vi "Config Input Settings.vi"(0 "VISA resource name":refnum<visa-resource-name>, 5 "Input (0: A)":u16(ring) items=["A", "B", "C", "D"], 7 "Compensation (0: Off)":i8(ring) items=["Off", "On", "Pause", "Reverse"], 9 "Scan Enable (F: Disable Scanning)":bool, 11 "error in (no error)":errorcluster, 12 "Curve Number (0)":dbl min=0.0 max=60.0 step=1.0) -> (4 "VISA resource name out":refnum<visa-resource-name>, 15 "error out":errorcluster)   [LabVIEW 2019, in "Lake Shore Cryotronics 340.lvlib"]
doc: "This VI configures the following settings for the 340 inputs:\nScan Enable, Compensation, and Curve Number.\nThe LSCI 340 Status - Busy.vi should be used after this vi to verify the instrument has finished processing the commands."
uses:
  Lake Shore Cryotronics 340.lvlib
panel:
  # "Enable Scanning\nDisable Scanning"
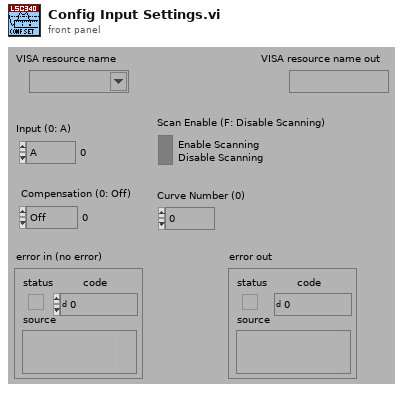
[diagram p1: front panel]
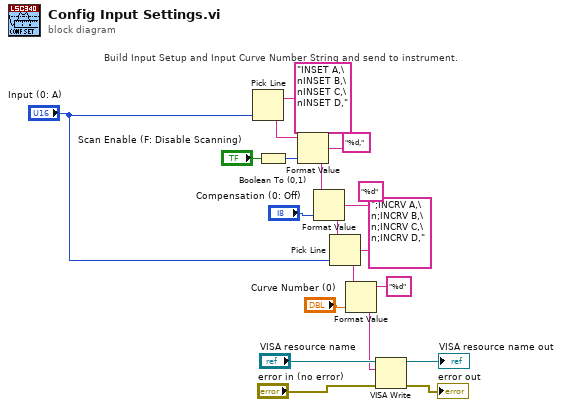
[diagram p0: block diagram]
diagram:
  # "Build Input Setup and Input Curve Number String and send to instrument."
  n1 = Pick Line(multi-line string="INSET A,\nINSET B,\nINSET C,\nINSET D,", line index="Input (0: A)") -> (output string=w9:string)  [unwired: 1 in]
  n2 = Boolean To (0,1)(Boolean="Scan Enable (F: Disable Scanning)") -> (0, 1=w10:i16)
  n3 = Format Value(string ("")=w9, format string="%d,", value (0)=w10) -> (output string=w8:string)
  n4 = Format Value(string ("")=w8, format string="%d", value (0)="Compensation (0: Off)") -> (output string=w7:string)
  n5 = Pick Line(string ("")=w7, multi-line string=";INCRV A,\n;INCRV B,\n;INCRV C,\n;INCRV D,", line index="Input (0: A)") -> (output string=w13:string)
  n6 = Format Value(string ("")=w13, format string="%d", value (0)="Curve Number (0)") -> (output string=w1:string)
  n7 = VISA Write(VISA resource name="VISA resource name", write buffer=w1, error in (no error)="error in (no error)") -> (VISA resource name out=→"VISA resource name out":refnum<visa-resource-name>, error out=→"error out":errorcluster)  [unwired: 1 out]
